vi "GPIO Number.vi"(4 "AI in":refnum<class "AI.lvclass">) -> (7 "GPIO #":T1=-1)   [LabVIEW 2020, in "CTI.lvlib" / "AI.lvclass"]
uses:
  AI.lvclass
  GPIO Number.ctl
  AI.lvclass/AI.ctl
  GPIO/GPIO.lvclass/GPIO.ctl
  GPIO/GPIO.lvclass
  CTI.lvlib
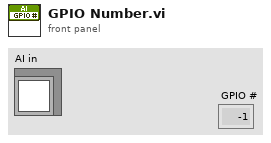
[diagram p1: front panel]
types:
  T1 = typedef "CTI.lvlib/GPIO Number.ctl" = i8
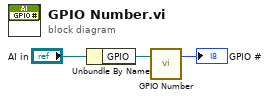
[diagram p0: block diagram]
diagram:
  n1 = Unbundle By Name("AI in") -> ("GPIO"=w2:refnum<class "GPIO.lvclass">)
  n2 = call "GPIO Number.vi"("GPIO in"=w2) -> ("GPIO #"=→"GPIO #":T1)  [unwired: 6 in]
